vi "Display.vi"(0 "VISA resource name":refnum<visa-resource-name>, 5 "Mode(F:Meter)":bool, 7 "Display(T:On)":bool=TRUE, 9 "String to write (National Instruments)":string="National Instruments", 11 "error in (no error)":errorcluster) -> (4 "VISA resource name out":refnum<visa-resource-name>, 15 "error out":errorcluster)   [LabVIEW 2012, in "Agilent 66XX Series.lvlib"]
doc: "This vi controls various issues concerning the display of the power supply. The display can either be turned on or off. There are also controls to determine what mode the instrument is operating in as well as a string input that can be written and displayed."
uses:
  <instrlib>/Agilent 66XX Series/Agilent 66XX Series.lvlib
panel:
  # "On"
  # "Off"
  # "User Text"
  # "Meter mode"
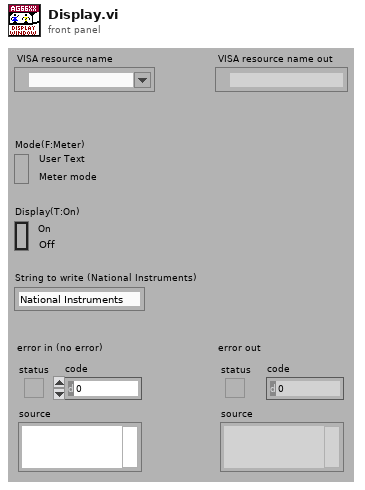
[diagram p1: front panel]
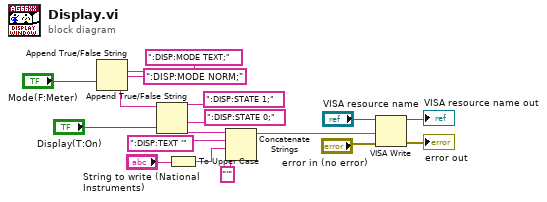
[diagram p0: block diagram]
diagram:
  n1 = Append True/False String(1:"Mode(F:Meter)", 2:":DISP:MODE NORM;", 3:":DISP:MODE TEXT;") -> (0:w7:string)  [unwired: 1 in]
  n2 = Append True/False String(1:"Display(T:On)", 2:":DISP:STATE 0;", 3:":DISP:STATE 1;", 4:w7) -> (0:w6:string)
  n3 = To Upper Case(1:"String to write (National Instruments)") -> (0:w1:string)
  n4 = Concatenate Strings(w6, ":DISP:TEXT '", w1, "'") -> (w5:string)
  n5 = VISA Write(VISA resource name="VISA resource name", write buffer=w5, error in (no error)="error in (no error)") -> (VISA resource name out=→"VISA resource name out":refnum<visa-resource-name>, error out=→"error out":errorcluster)  [unwired: 1 out]
